vi "BRig_dataExp_Audio_pattern_R.vi"() -> (2 "output_Audio_sp__R":i32)   [LabVIEW 2014]
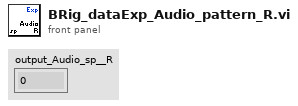
[diagram p1: front panel]
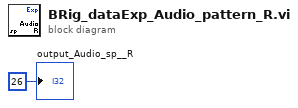
[diagram p0: block diagram]
diagram:
  "output_Audio_sp__R" <- 26 ("output_iBlock")
